vi "VHM-setSettings.vi"(8 "error in (no error)":errorcluster, 10 "settings":T1={"Start [hz]"=0, "Stop [hz]"=0, "sampleSize"=101} {"sampleSize" items=["101"=101, "201"=201, "401"=401, "601"=601, "801"=801, "1001"=1001]; "Stop [hz]" format="%.0p"; "Start [hz]" format="%.0p"}, 11 "VHM-VNA_Hardware_Manager in":refnum<class "VHM-VNA_Hardware_Manager.lvclass">) -> (0 "error out":errorcluster, 3 "VHM-VNA_Hardware_Manager out":refnum<class "VHM-VNA_Hardware_Manager.lvclass">)   [LabVIEW 2020, in "VHM-VNA_Hardware_Manager.lvlib" / "VHM-VNA_Hardware_Manager.lvclass"]
uses:
  VHM-VNA_Hardware_Manager.lvclass
  classes/vna-drivers/liteVNA/VD-settingsEasy.ctl
  classes/vna-drivers/liteVNA/VD-sampleSize.ctl
  VHM-VNA_Hardware_Manager.lvclass/VHM-VNA_Hardware_Manager.ctl
  classes/vna-drivers/liteVNA/VD-LV-LiteVNA.lvclass
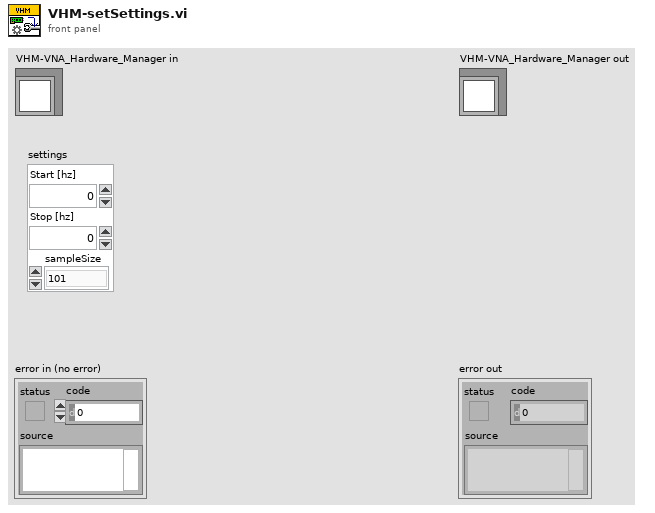
[diagram p1: front panel]
types:
  T1 = typedef "VD-LV-LiteVNA.lvclass/VD-settingsEasy.ctl" = cluster{"Start [hz]":u64, "Stop [hz]":u64, "sampleSize":T2}
  T2 = typedef "VD-LV-LiteVNA.lvclass/VD-sampleSize.ctl" = u16
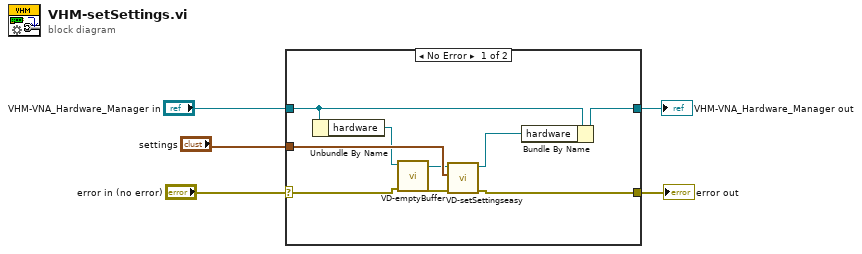
[diagram p0: block diagram]
diagram:
  n1 = case shown="No Error" "error in (no error)" {
    selector: "error in (no error)" -> [w6 w16]
    tunnel: [w10 w16] -> w4
    tunnel: [w13 w15] -> w2
    tunnel: "VHM-VNA_Hardware_Manager in" -> [w14 w15]
    tunnel: "settings" -> [w12 _]
    frame No Error {
      n2 = Unbundle By Name(w14) -> ("hardware"=w7:refnum<class "VD-LV-LiteVNA.lvclass">)
      n3 = call-dynamic "VD-emptyBuffer.vi"("error in (no error)"=w6, "VD-LV-LiteVNA in"=w7) -> ("error out"=w8:errorcluster, "VD-LV-LiteVNA out"=w9:refnum<class "VD-LV-LiteVNA.lvclass">)  [unwired: 5 in, 3 out]
      n4 = call "VD-setSettingseasy.vi"("error in (no error)"=w8, "settings"=w12, "VD-LV-LiteVNA in"=w9) -> ("error out"=w10:errorcluster, "VD-LV-LiteVNA out"=w11:refnum<class "VD-LV-LiteVNA.lvclass">)  [unwired: 7 in]
      n5 = Bundle By Name(cluster=w14, "hardware"=w11) -> (w13:refnum<class "VHM-VNA_Hardware_Manager.lvclass">)
    }
    frame Error {
    }
  }
  "error out" <- w4
  "VHM-VNA_Hardware_Manager out" <- w2
